vi "ReaderWriter-EndpointURL.vi"(8 "CTR ID #":i32, 9 "DAQ Endpoint":string, 10 "CTR IR Addr":string, 11 "DAQ IP Addr":string) -> (0 "DAQ Endpoint":string="CTR001", 1 "CTR Endpoint":string, 2 "CTR URL":string, 3 "DAQ URL":string)   [LabVIEW 2024]
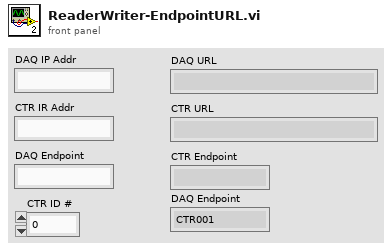
[diagram p1: front panel]
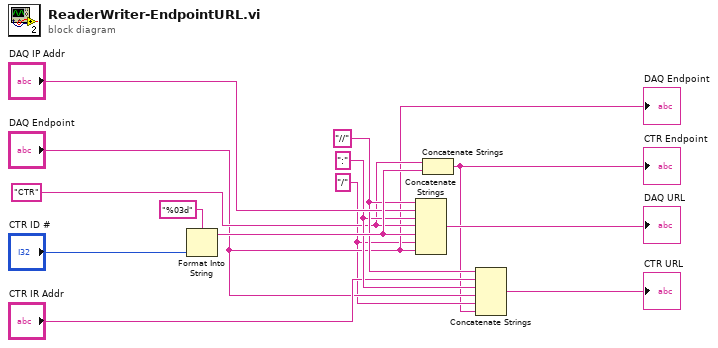
[diagram p0: block diagram]
diagram:
  w5 = "CTR" ("string")
  w6 = ":" ("string")
  w7 = "//" ("string")
  w2 = "/" ("string")
  n1 = Format Into String(format string="%03d", "CTR ID #") -> (resulting string=w13:string)  [unwired: 2 in, 1 out]
  n2 = Concatenate Strings(w7, "DAQ IP Addr", w6, w5, w13, w2, "DAQ Endpoint") -> (→"DAQ URL":string)
  n3 = Concatenate Strings(w5, w13) -> (w1:string)
  "CTR Endpoint" <- w1
  n4 = Concatenate Strings(w7, "CTR IR Addr", w6, "DAQ Endpoint", w2, w1) -> (→"CTR URL":string)
  "DAQ Endpoint" <- "DAQ Endpoint"
